vi "Measure.vi"(11 "DMMSession":refnum<k15>) -> (0 "error out":errorcluster)   [LabVIEW 2019]
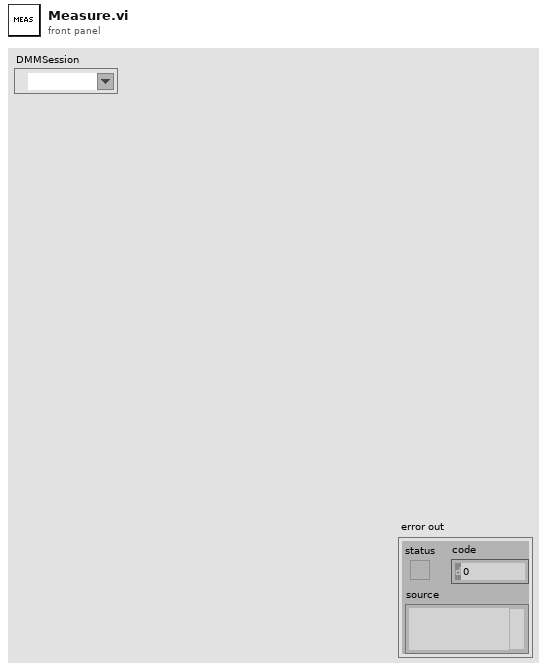
[diagram p1: front panel]
types:
  T1 = typedef "HVC5.lvlib/HVC5.lvclass/measurementservice_DMMConfigResponse_Data.ctl" = cluster{"DMMFunction":i32, "DMMResolution":sgl, "DMMRange":sgl, "DMMSampleCount":i32, "DMMApertureTimeUnit":i32, "DMMApertureTime":sgl, "DMMNumberofAverages":i32, "DMMAutoZero":i32, "DMMADCCalibration":i32, "DMMSettleTime":sgl, "error":T2}
  T2 = typedef "HVC5.lvlib/HVC5.lvclass/measurementservice_ErrorOut_Data.ctl" = cluster{"errCode":i32, "errMessage":string}
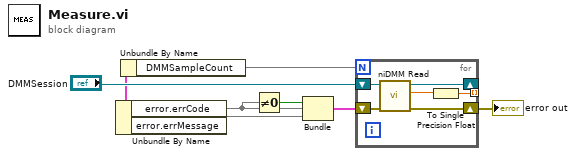
[diagram p0: block diagram]
diagram:
  n1 = Unbundle By Name() -> (w6:T1, "DMMSampleCount"=w7)
  n2 = Unbundle By Name(w6) -> ("error.errCode"=w2, "error.errMessage"=w4)
  n3 = Not Equal To 0?(x=w2) -> (x != 0?=w1:bool)
  n4 = Bundle(w1, "errCode"=w2, "errMessage"=w4) -> (w3:cluster{bool, "errCode":void, "errMessage":void}, w5:cluster{bool, "errCode":void, "errMessage":void})
  n5 = for {
    N: w7 -> [_]
    tunnel: [w11] -> w9 mode=indexing
    shift-right: [w15] -> w10
    shift-left: w3 -> [w14]
    shift-right: [w16] -> _
    shift-left: "DMMSession" -> [w13]
    n6 = call <instrlib>:"niDMM Read.vi"("error in (no error)"=w14, "instrument handle"=w13) -> ("error out"=w15:errorcluster, "Measurement"=w12:dbl, "instrument handle out"=w16:refnum<k15>)  [unwired: 7 in]
    n7 = To Single Precision Float(number=w12) -> (single precision float=w11:sgl)
  }
  "error out" <- w10
